vi "Moment Score.vi"(11 "Moment Factor":dbl) -> (3 "Score":dbl)   [LabVIEW 2025]
doc: "Calculate a score based on moment of inertia. There are many forms and this VI uses a normalized form that is more stable and is referred to as Type Factor."
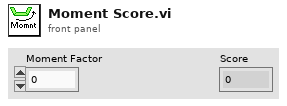
[diagram p1: front panel]
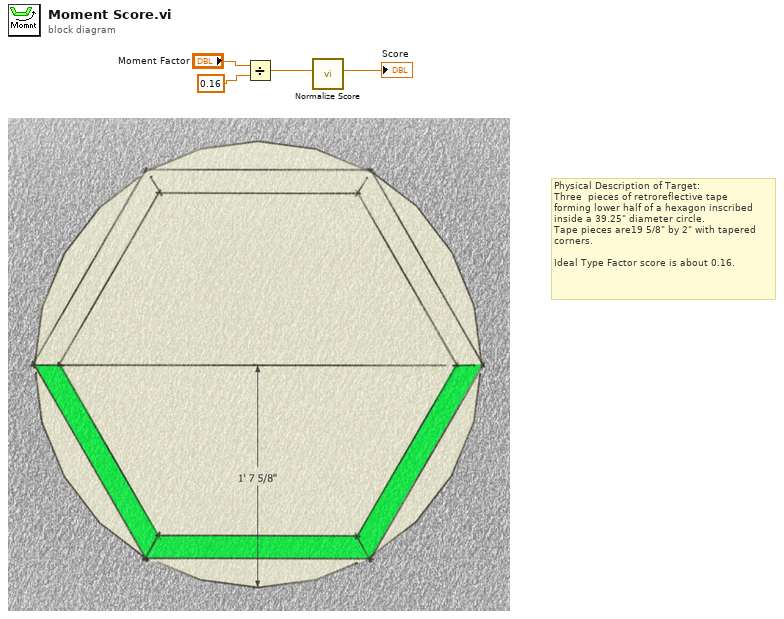
[diagram p0: block diagram]
diagram:
  # "Physical Description of Target:\nThree  pieces of retroreflective tape\nforming lower half of a hexagon inscribed\ninside a 39.25\" diameter circle.\nTape pieces are19 5/8\" by 2\" with tapered\ncorners.\n\nIdeal Type Factor score is about 0.16."
  n1 = Divide(x="Moment Factor", y=0.16 ("length")) -> (x/y=w3:dbl)
  n2 = call "Normalize Score.vi"("Value"=w3) -> ("Score"=→"Score":dbl)  [unwired: 10 in]
